vi "Mask Applicator.vi"(3 "ROI Different":bool[](array[boolean]), 5 "ROI In":T3[](array[typedef]) {"Contours"."Type" items=["No Selection", "Point", "Line", "Rectangle", "Oval", "Polygon", "Freehand Region", "Annulus", "Unused2", "Unused3", "Broken Line", "Freehand Line", "Rotated Rectangle"]}, 6 "Cluster":T1={"Rectangle Color"=16711680, "Text Color"=6618880, "Fill Color"=16776960}, 7 "ROI Number":u16, 8 "ROI List In":string[](array[string]), 9 "Event Coordinates":i32[](array[numeric]), 10 "Event Type":i32, 11 "Image Mask":T2) -> (0 "error out":errorcluster, 2 "ROI Out":T3[](array[typedef]) {"Contours"."Type" items=["No Selection", "Point", "Line", "Rectangle", "Oval", "Polygon", "Freehand Region", "Annulus", "Unused2", "Unused3", "Broken Line", "Freehand Line", "Rotated Rectangle"]})   [LabVIEW 2015]
uses:
  <vilib>/vision/Image Controls.llb/IMAQ Image.ctl
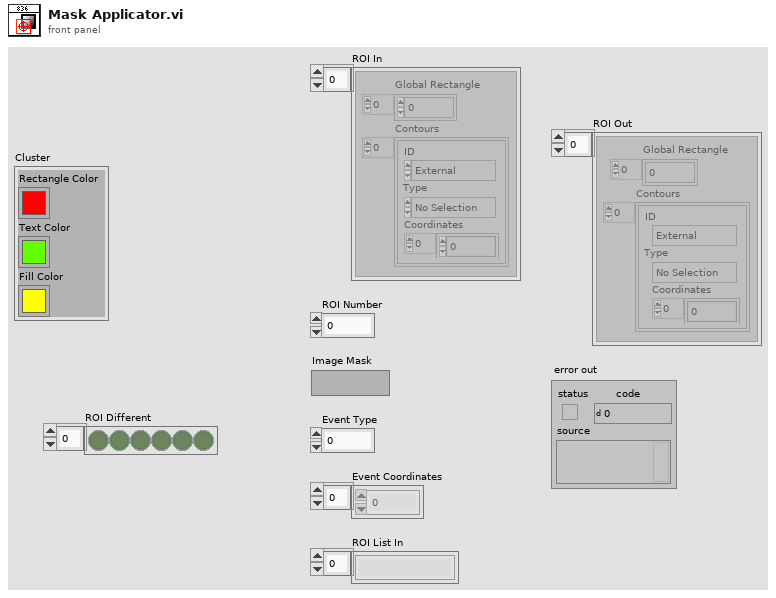
[diagram p1: front panel]
types:
  T1 = cluster{"Rectangle Color":u32, "Text Color":u32, "Fill Color":u32}
  T2 = typedef "IMAQ Image.ctl" = refnum<image>
  T3 = typedef "ROI Descriptor" = cluster{"Global Rectangle":i32[], "Contours":cluster{"ID":enum32{"External", "Internal"}, "Type":u32, "Coordinates":i32[]}[]}
  T4 = typedef "IMAQ Rectangle" = cluster{"Left":i32, "Top":i32, "Right":i32, "Bottom":i32, "Rotation":dbl}
  T5 = cluster{"[0]":i32, "[1]":i32, "[2]":i32, "[3]":i32}
  T6 = cluster{"Event Coordinates[0]":i32, "Event Coordinates[1]":i32, "Event Coordinates[2]":i32, "Event Coordinates[3]":i32}
  T7 = cluster{"Event Coordinates":cluster{"Event Coordinates[0]":i32, "Event Coordinates[1]":i32, "Event Coordinates[2]":i32, "Event Coordinates[3]":i32}, dbl}
  T8 = cluster{"Event Coordinates[0]":i32, "Event Coordinates[1]":i32}
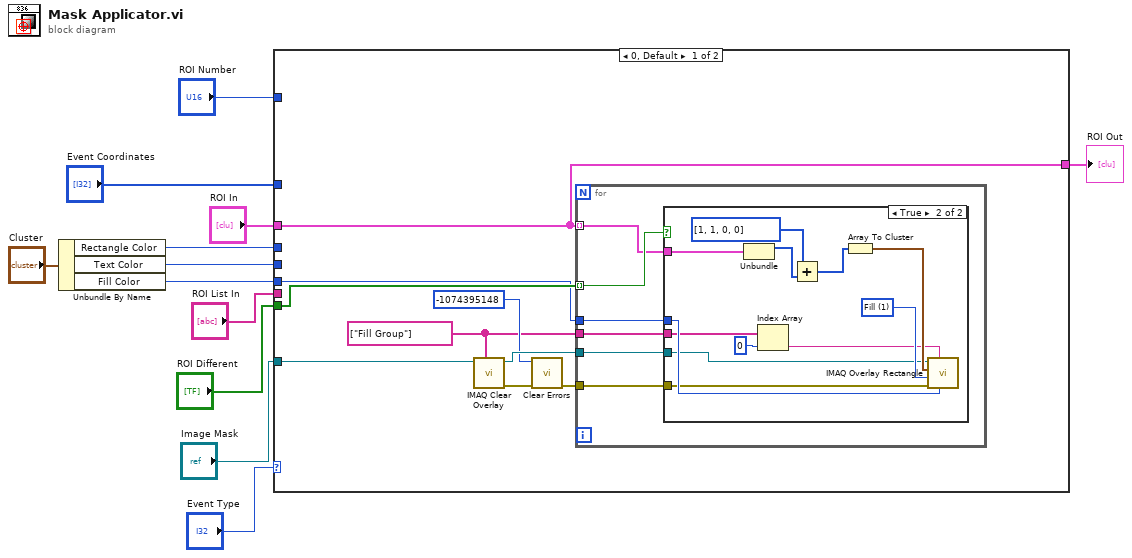
[diagram p0: block diagram]
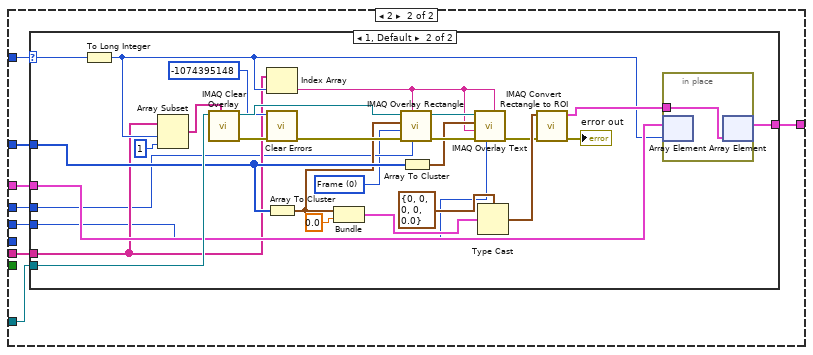
[diagram p3: hidden frame]
diagram:
  n1 = Unbundle By Name("Cluster") -> ("Rectangle Color"=w4:u32, "Text Color"=w3:u32, "Fill Color"=w2:u32)
  n2 = case shown="0, Default" "Event Type" {
    tunnel: "Event Coordinates" -> [_ w46]
    tunnel: "Image Mask" -> [w18 w47]
    tunnel: "ROI List In" -> [_ w45]
    tunnel: "ROI In" -> [w19 w44]
    tunnel: [w19 w43] -> w9
    tunnel: w4 -> [_ w42]
    tunnel: w3 -> [_ w41]
    tunnel: "ROI Number" -> [_ w40]
    tunnel: w2 -> [w20 _]
    tunnel: "ROI Different" -> [w21 _]
    frame 0, Default {
      w13 = string[] ["Fill Group"] ("Groups")
      n3 = call "IMAQ Clear Overlay"("Groups"=w13, "Image"=w18) -> ("error out"=w15:errorcluster, "Image Out"=w17:T2)  [unwired: 8 in]
      n4 = call <vilib>:"Clear Errors.vi"("error in (no error)"=w15, "specific error code to clear (0: all)"=-1074395148) -> ("error out"=w14:errorcluster)  [unwired: 4 in, 1 out]
      n5 = for {
        tunnel: w21 -> [w27] mode=indexing
        tunnel: w17 -> [w26]
        tunnel: w20 -> [w25]
        tunnel: w19 -> [w24] mode=indexing
        tunnel: w14 -> [w23]
        tunnel: w13 -> [w22]
        n6 = case shown="True" w27 {
          tunnel: w26 -> [_ w35]
          tunnel: w25 -> [_ w38]
          tunnel: w24 -> [_ w37]
          tunnel: w23 -> [_ w34]
          tunnel: w22 -> [_ w33]
          frame False {
          }
          frame True {
            w39 = u32 1 items=["Frame", "Fill", "Highlight"] ("Drawing Mode (Frame)")
            n7 = Unbundle(w37) -> ("Global Rectangle"=w30:i32[])  [unwired: 1 out]
            n8 = Index Array(array=w33, index=0) -> (element=w31:string)
            n9 = Add(x=i32[] [1, 1, 0, 0], y=w30) -> (x+y=w28:i32[])
            n10 = Array To Cluster(array=w28) -> (cluster=w36:T5)
            n11 = call "IMAQ Overlay Rectangle"("Color"=w38, "Group"=w31, "error in (no error)"=w34, "Drawing Mode (Frame)"=w39, "Rectangle"=w36, "Image"=w35) -> ()  [unwired: 4 in, 2 out]
          }
        }
      }
    }
    frame 2 {
      n12 = case shown="1, Default" w40 {
        selector: w40 -> [_ w71]
        tunnel: w47 -> [_ w76]
        tunnel: w46 -> [_ w64]
        tunnel: w45 -> [_ w52]
        tunnel: w44 -> [w48 w57]
        tunnel: [w48 w55] -> w43
        tunnel: w42 -> [_ w51]
        tunnel: w41 -> [_ w50]
        frame 0 {
        }
        frame 1, Default {
          w49 = u32 0 items=["Frame", "Fill", "Highlight"] ("Drawing Mode (Frame)")
          n13 = To Long Integer(number=w71) -> (32bit integer=w56:i32)
          n14 = Array Subset(array=w52, index=w56, length=1) -> (w68:string[])
          n15 = call "IMAQ Clear Overlay"("Groups"=w68, "Image"=w76) -> ("error out"=w67:errorcluster, "Image Out"=w75:T2)  [unwired: 8 in]
          n16 = Index Array(array=w52, index=w56) -> (element=w70:string)
          n17 = call <vilib>:"Clear Errors.vi"("error in (no error)"=w67, "specific error code to clear (0: all)"=-1074395148) -> ("error out"=w66:errorcluster)  [unwired: 4 in, 1 out]
          n18 = Array To Cluster(array=w64) -> (cluster=w61:T6)
          n19 = Bundle("Event Coordinates"=w61, 0.0) -> (w63:T7)  [unwired: 1 in]
          n20 = call "IMAQ Overlay Rectangle"("Color"=w51, "Group"=w70, "error in (no error)"=w66, "Drawing Mode (Frame)"=w49, "Rectangle"=w61, "Image"=w75) -> ("error out"=w74:errorcluster, "Image Out"=w73:T2)  [unwired: 4 in]
          n21 = Array To Cluster(array=w64) -> (cluster=w72:T8)
          n22 = call "IMAQ Overlay Text"("Group"=w70, "Text Color (black)"=w50, "error in (no error)"=w74, "String"=w70, "Origin"=w72, "Image"=w73) -> ("error out"=w54:errorcluster)  [unwired: 4 in, 1 out]
          n23 = Type Cast(type=T4 {"Left"=0, "Top"=0, "Right"=0, "Bottom"=0, "Rotation"=0.0} ("Rectangle"), x=w63) -> (*(type *) &x=w60:T4)
          n24 = call "IMAQ Convert Rectangle to ROI"("error in (no error)"=w54, "Rectangle"=w60) -> ("error out"=→"error out":errorcluster, "ROI Descriptor"=w58:T3)  [unwired: 7 in]
          n25 = in-place {
            in-place-border: w58 -> [w77]
            n26 = in-place-array #1(w57, w56) -> ()  [unwired: 1 out]
            n27 = in-place-array #1(w77) -> (w55:T3[])  [unwired: 1 out]
          }
        }
      }
    }
  }
  "ROI Out" <- w9
